vi "Run Framework.vi"(5 "components directory":path, 7 "framework options":T14={"FIFO Options"={"Infinite Timeouts"=FALSE}, "Thread Options"={"Show FP On Call"=TRUE, "Close FP After Call"=TRUE, "Allow Debugging"=TRUE, "Restart On Error"=FALSE}, "Plugin Options"={"Default Components"=TRUE}, "Performance Options"={"Measure Period"=TRUE, "Measure Rx/Tx Duration"=TRUE}}, 8 "error in (no error)":errorcluster, 9 "thread settings":cluster{"Processor":i32, "Priority":i32}={"Processor"=-2, "Priority"=100}, 10 "framework configuration":T2, 11 "user interface pointers (null)":T1) -> (0 "error out":errorcluster)   [LabVIEW 2017]
uses:
  Builds/Data Sharing Framework/Current/Core/DSF Core.lvlibp/Classes/Framework/Framework Options.ctl
  Builds/Data Sharing Framework/Current/Core/DSF Core.lvlibp/Typedefs/DSF FIFO Options.ctl
  Builds/Data Sharing Framework/Current/Core/DSF Core.lvlibp/Classes/Thread/Thread Options.ctl
  Builds/Data Sharing Framework/Current/Core/DSF Core.lvlibp/Typedefs/DSF Plugin Options.ctl
  Builds/Data Sharing Framework/Current/Core/DSF Core.lvlibp/Typedefs/DSF Performance Options.ctl
  Builds/Data Sharing Framework/Current/Core/DSF Core.lvlibp/Typedefs/DSF Engine Framework Configuration.ctl
  Builds/Data Sharing Framework/Current/Core/DSF Core.lvlibp/Typedefs/DSF Engine Plugin Configuration.ctl
  Builds/Data Sharing Framework/Current/Core/DSF Core.lvlibp/Typedefs/DSF Timing Info.ctl
  Builds/Data Sharing Framework/Current/Core/DSF Core.lvlibp/Typedefs/DSF Engine Plugin Thread Configuration.ctl
  Builds/Data Sharing Framework/Current/Core/DSF Core.lvlibp/Typedefs/DSF Settings Info.ctl
  Builds/Data Sharing Framework/Current/Core/DSF Core.lvlibp/Typedefs/DSF Engine Transfer Group Configuration.ctl
  Builds/Data Sharing Framework/Current/Core/DSF Core.lvlibp/Typedefs/DSF Direction.ctl
  Builds/Data Sharing Framework/Current/Core/DSF Core.lvlibp/Typedefs/DSF Engine Transfer Configuration.ctl
  Builds/Data Sharing Framework/Current/Core/DSF Core.lvlibp/Typedefs/DSF Byte Order.ctl
  Builds/Data Sharing Framework/Current/Core/DSF Core.lvlibp/Typedefs/DSF Engine Channel Configuration.ctl
  Builds/Data Sharing Framework/Current/Core/DSF Core.lvlibp/Typedefs/DSF Data Type.ctl
  Builds/Data Sharing Framework/Current/Core/DSF Core.lvlibp/Typedefs/DSF Timeout Behavior.ctl
  SubVIs/UI Pointers.ctl
  <vilib>/NI/Memory Manager/Classes/Pointer/Pointer.lvclass
  <vilib>/NI/Memory Manager/Classes/Pointer/Pointer.lvclass/Pointer.ctl
  <vilib>/Platform/TimedLoop/XDataNode/timing_clust.ctl
  <vilib>/Platform/TimedLoop/XDataNode/nitl_modes.ctl
  <vilib>/Platform/TimedLoop/XDataNode/wakeup.ctl
  <vilib>/NI/Memory Manager/Classes/Pointer/Write U32.vi
  <vilib>/NI/Memory Manager/Classes/Pointer/Read U32.vi
  <vilib>/NI/Memory Manager/Classes/Pointer/Read I32.vi
  <vilib>/NI/Memory Manager/Classes/Pointer/Read Bool.vi
  <vilib>/NI/Memory Manager/Classes/Pointer/Write Bool.vi
  <vilib>/NI/Memory Manager/Classes/Pointer/Write I32.vi
  <vilib>/NI/Memory Manager/Classes/Pointer/Set Address.vi
  <vilib>/NI/Memory Manager/Classes/Pointer/Set Size.vi
  <vilib>/NI/Memory Manager/Classes/Pointer/Set Internal.vi
  <vilib>/NI/Memory Manager/Classes/Pointer/Check Null Pointer.vi
  <vilib>/NI/Memory Manager/Classes/Pointer/Clear (No Check).vi
  <vilib>/NI/Memory Manager/Classes/Pointer/Check Length.vi
  <vilib>/NI/Memory Manager/Classes/Pointer/Write (No Check).vi
  <vilib>/NI/Memory Manager/Classes/Pointer/Write (No Check) U32.vi
  <vilib>/NI/Memory Manager/Classes/Pointer/Check Move.vi
  <vilib>/NI/Memory Manager/Classes/Pointer/Read (No Check).vi
  <vilib>/NI/Memory Manager/Classes/Pointer/Read (No Check) U32.vi
  <vilib>/NI/Memory Manager/Classes/Pointer/Read (No Check) I32.vi
  <vilib>/NI/Memory Manager/Classes/Pointer/Read (No Check) Bool.vi
  <vilib>/NI/Memory Manager/Classes/Pointer/Write (No Check) Bool.vi
  <vilib>/NI/Memory Manager/Classes/Pointer/Write (No Check) I32.vi
  <vilib>/NI/Memory Manager/Classes/Pointer/Get Internal.vi
  <vilib>/NI/Memory Manager/Classes/Pointer/Errors.vi
  <vilib>/NI/Memory Manager/Classes/Pointer/Zone.vi
  <vilib>/NI/Memory Manager/Classes/Pointer/Null Pointer.vi
  <vilib>/NI/Memory Manager/Classes/Pointer/Check Bounds (Pointer).vi
  <vilib>/NI/Memory Manager/Classes/Pointer/Check Count.vi
  <vilib>/NI/Memory Manager/Classes/Pointer/Check Bounds (Power of 2).vi
  <vilib>/NI/Memory Manager/Classes/Pointer/Create Error.vi
  <vilib>/NI/Memory Manager/Classes/Pointer/Out of Bounds.vi
  <vilib>/NI/Memory Manager/Classes/Pointer/Check Bounds.vi
  <vilib>/NI/Memory Manager/Constants/Constants.vi
  <vilib>/NI/Memory Manager/Constants/Library Name.vi
  <vilib>/NI/Memory Manager/Classes/Pointer/Pointer Error Info.vi
  <vilib>/NI/Memory Manager/Constants/Pointer Class Name.vi
  <vilib>/NI/Memory Manager/Classes/Pointer/Write Pointer Size to Error.vi
  <vilib>/NI/Memory Manager/Classes/Pointer/Check Bounds (Buffer).vi
  <vilib>/NI/Memory Manager/Classes/Pointer/Buffer Underflow.vi
  <vilib>/NI/Memory Manager/VIs/New Error Cluster.vi
  <vilib>/NI/Memory Manager/VIs/New Error Cluster (512B).vi
  <vilib>/NI/Memory Manager/VIs/Set Error Status.vi
  <vilib>/NI/Memory Manager/VIs/Set Error Code.vi
  <vilib>/NI/Memory Manager/VIs/Set Error Source.vi
  <vilib>/NI/Memory Manager/VIs/Write String to Source.vi
  <vilib>/NI/Memory Manager/VIs/Write Numeric to Source.vi
  <vilib>/NI/Memory Manager/VIs/Write Numeric Scalar to Source (Base10 U64).vi
  Builds/Data Sharing Framework/Current/Core/DSF Core.lvlibp/Classes/Framework/Framework.lvclass
  <vilib>/platform/TimedLoop/XDataNode/XDataNode.xnode
  <vilib>/Platform/TimedLoop/XDataNode/XDNodeRunTimeDep.lvlib
  Builds/Data Sharing Framework/Current/Core/DSF Core.lvlibp
  Builds/Data Sharing Framework/Current/Core/DSF Core.lvlibp/Classes/Thread/Thread.lvclass
panel:
  out "actual frequency":u32 format="%.0pHz"
  in  "target frequency":u32=100 format="%.0pHz"
  out "iteration":i32
  in  "stop":bool
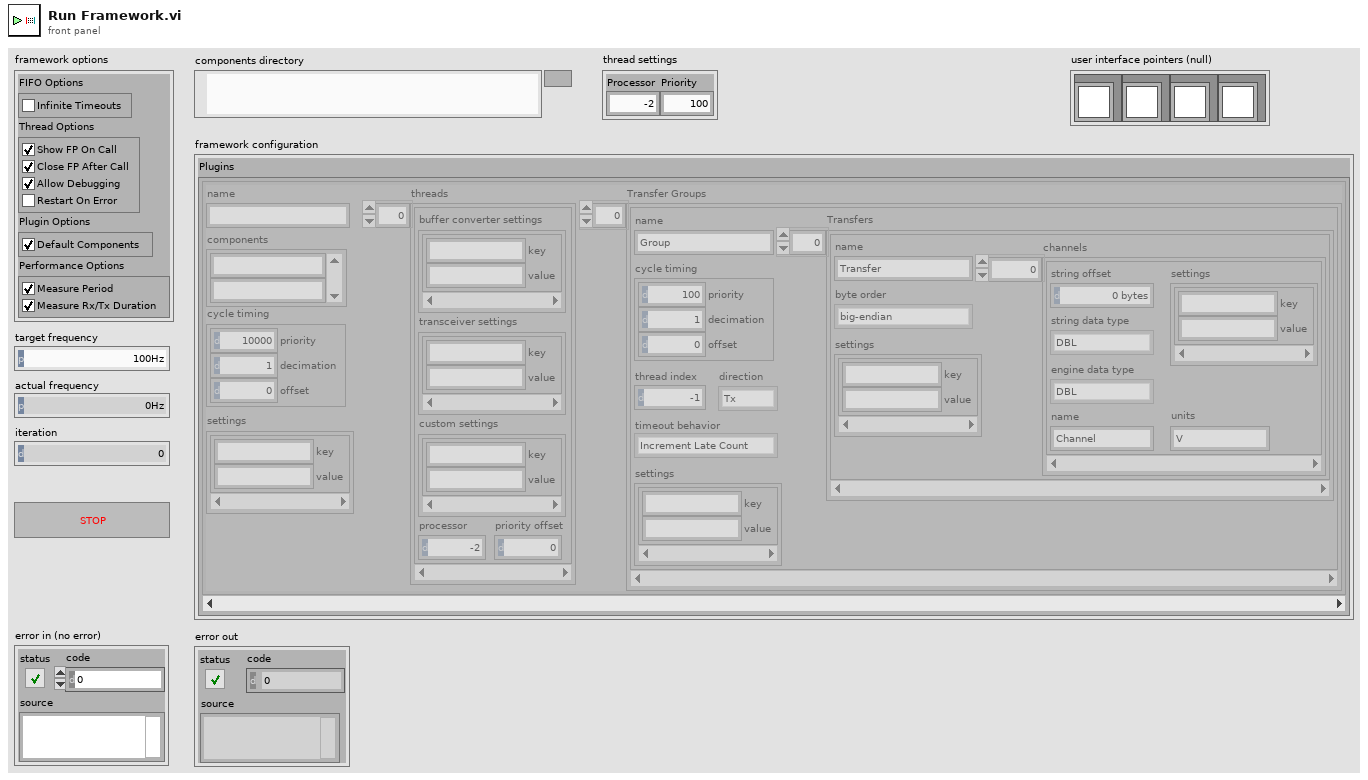
[diagram p1: front panel]
types:
  T1 = typedef "UI Pointers.ctl" = cluster{"Stop":refnum<class "Pointer.lvclass">, "Target Period":refnum<class "Pointer.lvclass">, "Actual Period":refnum<class "Pointer.lvclass">, "Iteration":refnum<class "Pointer.lvclass">}
  T2 = typedef "DSF Core.lvlibp/DSF Engine Framework Configuration.ctl" = cluster{"Plugins":T3[]}
  T3 = typedef "DSF Core.lvlibp/DSF Engine Plugin Configuration.ctl" = cluster{"name":string, "components":string[], "cycle timing":T4, "threads":T5[], "Transfer Groups":T7[], "settings":T6}
  T4 = typedef "DSF Core.lvlibp/DSF Timing Info.ctl" = cluster{"priority":u64, "decimation":u64, "offset":u64}
  T5 = typedef "DSF Core.lvlibp/DSF Engine Plugin Thread Configuration.ctl" = cluster{"buffer converter settings":T6, "transceiver settings":T6, "custom settings":T6, "processor":i32, "priority offset":i16}
  T6 = typedef "DSF Core.lvlibp/DSF Settings Info.ctl" = cluster{"key":string, "value":string}[]
  T7 = typedef "DSF Core.lvlibp/DSF Engine Transfer Group Configuration.ctl" = cluster{"name":string, "direction":T8, "cycle timing":T4, "thread index":i32, "settings":T6, "Transfers":T9[], "timeout behavior":T13}
  T8 = typedef "DSF Core.lvlibp/DSF Direction.ctl" = enum8{"Tx", "Rx"}
  T9 = typedef "DSF Core.lvlibp/DSF Engine Transfer Configuration.ctl" = cluster{"name":string, "byte order":T10, "settings":T6, "channels":T11[]}
  T10 = typedef "DSF Core.lvlibp/DSF Byte Order.ctl" = enum8{"big-endian", "little-endian"}
  T11 = typedef "DSF Core.lvlibp/DSF Engine Channel Configuration.ctl" = cluster{"string offset":u64, "string data type":T12, "engine data type":T12, "name":string, "settings":T6, "units":string}
  T12 = typedef "DSF Core.lvlibp/DSF Data Type.ctl" = enum8{"Bool", "SGL", "DBL", "I8", "I16", "I32", "I64", "U8", "U16", "U32", "U64"}
  T13 = typedef "DSF Core.lvlibp/DSF Timeout Behavior.ctl" = enum8{"Increment Late Count", "Throw Error"}
  T14 = typedef "DSF Core.lvlibp/Framework.lvclass/Framework Options.ctl" = cluster{"FIFO Options":T15, "Thread Options":T16, "Plugin Options":T17, "Performance Options":T18}
  T15 = typedef "DSF Core.lvlibp/Framework.lvclass/DSF FIFO Options.ctl" = cluster{"Infinite Timeouts":bool}
  T16 = typedef "DSF Core.lvlibp/Thread.lvclass/Thread Options.ctl" = cluster{"Show FP On Call":bool, "Close FP After Call":bool, "Allow Debugging":bool, "Restart On Error":bool}
  T17 = typedef "DSF Core.lvlibp/Framework.lvclass/DSF Plugin Options.ctl" = cluster{"Default Components":bool}
  T18 = typedef "DSF Core.lvlibp/DSF Performance Options.ctl" = cluster{"Measure Period":bool, "Measure Rx/Tx Duration":bool}
  T19 = typedef "XDNodeRunTimeDep.lvlib/timing_clust.ctl" = cluster{"Expected End [f-1]":u64, "Actual End [f-1]":u64, "Finished Late? [f-1]":bool, "Expected End [i-1]":u64, "Actual End [i-1]":u64, "Finished Late? [i-1]":bool, "Expected Start [i]":u64, "Actual Start [i]":u64, "Expected Start [f]":u64, "Actual Start [f]":u64, "Source Name":string, "Structure Name":string, "Period":i64, "Deadline":i64, "Offset":i64, "Start":i64, "Priority":i32, "Timeout":i32, "Mode":T20, "Wakeup Reason":T21, "Error":errorcluster, "Source Type":string, "Secondary Source Type":string, "Global End Time":u64, "Global Start Time":u64, "Frame Duration":u64, "Iteration Duration":u64, "Assigned CPU":i32, "I/O Scan Engine Mode":u32}
  T20 = typedef "XDNodeRunTimeDep.lvlib/nitl_modes.ctl" = enum32{"No Change", "Process missed periods, maintain original phase", "Discard missed periods, maintain original phase", "Process missed periods, ignore original phase", "Discard missed periods, ignore original phase"}
  T21 = typedef "XDNodeRunTimeDep.lvlib/wakeup.ctl" = enum32{"Normal", "Aborted", "Asynchronous wakeup", "Timing source error", "Timed loop error", "Timeout"}
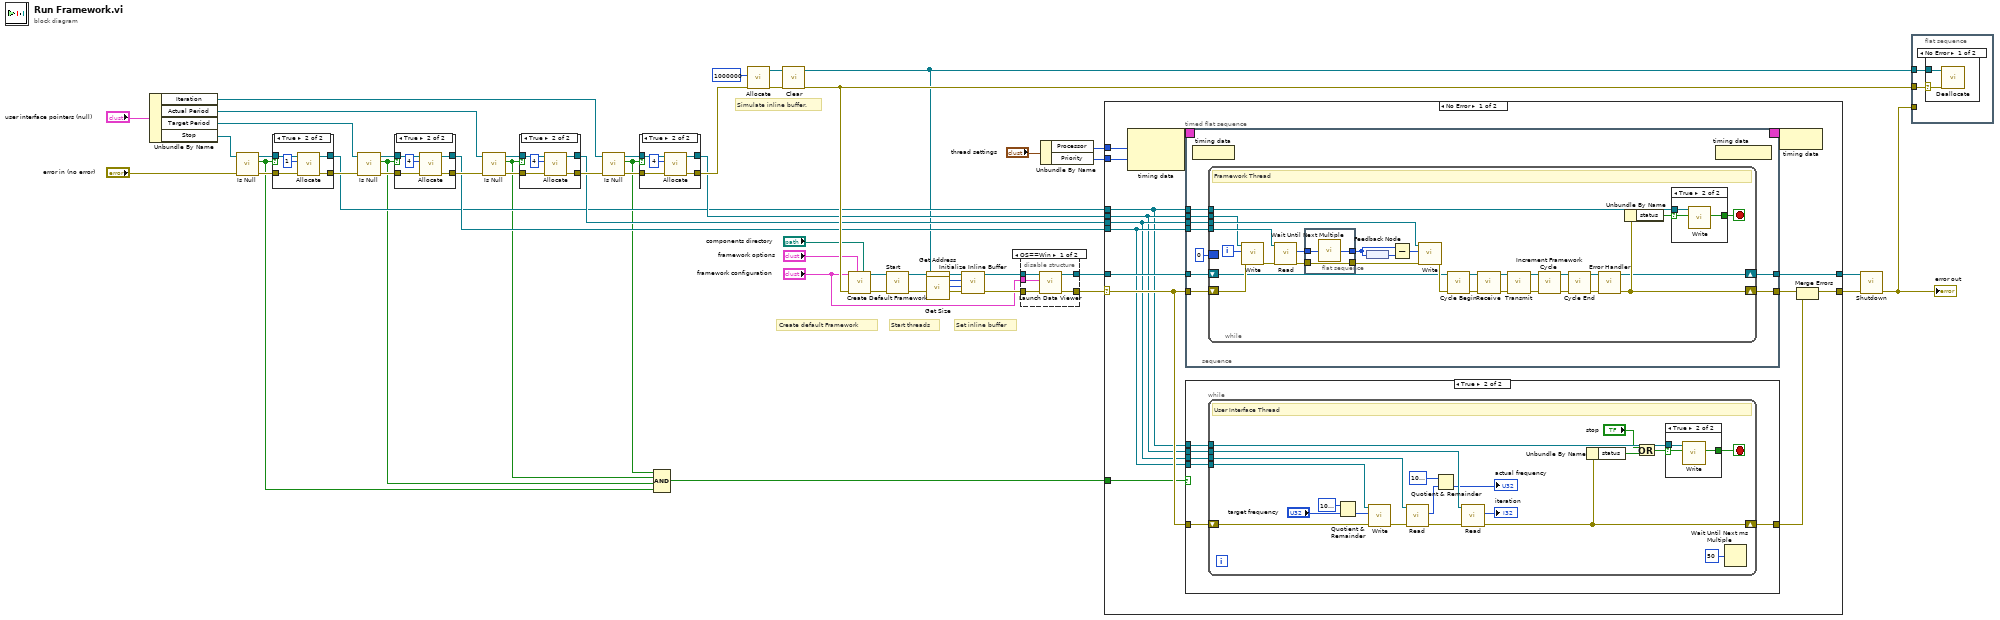
[diagram p0: block diagram]
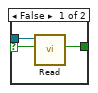
[diagram p5: hidden frame]
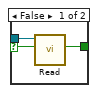
[diagram p6: hidden frame]
diagram:
  # "Set inline buffer"
  # "Start threads"
  # "Create default Framework"
  # "Simulate inline buffer."
  n1 = Unbundle By Name("user interface pointers (null)") -> ("Iteration"=w18:refnum<class "Pointer.lvclass">, "Actual Period"=w22:refnum<class "Pointer.lvclass">, "Target Period"=w26:refnum<class "Pointer.lvclass">, "Stop"=w32:refnum<class "Pointer.lvclass">)
  n2 = call <vilib>:"Is Null.vi"("error in (no error)"="error in (no error)", "Pointer in"=w32) -> ("error out"=w30:errorcluster, "null?"=w5:bool, "Pointer out"=w31:refnum<class "Pointer.lvclass">)  [unwired: 7 in]
  n3 = case shown="True" w5 {
    tunnel: w31 -> [w53 w57]
    tunnel: w30 -> [w52 w56]
    tunnel: [w53 w55] -> w11
    tunnel: [w52 w54] -> w27
    frame False {
    }
    frame True {
      n4 = call <vilib>:"Allocate.vi"("error in (no error)"=w56, "size"=u64 1, "Pointer type"=w57) -> ("error out"=w54:errorcluster, "Pointer out"=w55:refnum<class "Pointer.lvclass">)  [unwired: 7 in]
    }
  }
  n5 = call <vilib>:"Is Null.vi"("error in (no error)"=w27, "Pointer in"=w26) -> ("error out"=w28:errorcluster, "null?"=w4:bool, "Pointer out"=w29:refnum<class "Pointer.lvclass">)  [unwired: 7 in]
  n6 = case shown="True" w4 {
    tunnel: w29 -> [w60 w64]
    tunnel: w28 -> [w59 w63]
    tunnel: [w60 w62] -> w16
    tunnel: [w59 w61] -> w23
    frame False {
    }
    frame True {
      n7 = call <vilib>:"Allocate.vi"("error in (no error)"=w63, "size"=u64 4, "Pointer type"=w64) -> ("error out"=w61:errorcluster, "Pointer out"=w62:refnum<class "Pointer.lvclass">)  [unwired: 7 in]
    }
  }
  n8 = call <vilib>:"Is Null.vi"("error in (no error)"=w23, "Pointer in"=w22) -> ("error out"=w24:errorcluster, "null?"=w3:bool, "Pointer out"=w25:refnum<class "Pointer.lvclass">)  [unwired: 7 in]
  n9 = case shown="True" w3 {
    tunnel: w25 -> [w67 w71]
    tunnel: w24 -> [w66 w70]
    tunnel: [w67 w69] -> w13
    tunnel: [w66 w68] -> w19
    frame False {
    }
    frame True {
      n10 = call <vilib>:"Allocate.vi"("error in (no error)"=w70, "size"=u64 4, "Pointer type"=w71) -> ("error out"=w68:errorcluster, "Pointer out"=w69:refnum<class "Pointer.lvclass">)  [unwired: 7 in]
    }
  }
  n11 = call <vilib>:"Is Null.vi"("error in (no error)"=w19, "Pointer in"=w18) -> ("error out"=w20:errorcluster, "null?"=w2:bool, "Pointer out"=w21:refnum<class "Pointer.lvclass">)  [unwired: 7 in]
  n12 = case shown="True" w2 {
    tunnel: w21 -> [w74 w78]
    tunnel: w20 -> [w73 w77]
    tunnel: [w74 w76] -> w14
    tunnel: [w73 w75] -> w17
    frame False {
    }
    frame True {
      n13 = call <vilib>:"Allocate.vi"("error in (no error)"=w77, "size"=u64 4, "Pointer type"=w78) -> ("error out"=w75:errorcluster, "Pointer out"=w76:refnum<class "Pointer.lvclass">)  [unwired: 7 in]
    }
  }
  n14 = Compound Arithmetic op=AND(w2, w3, w4, w5) -> (w1:bool)
  n15 = call <vilib>:"Allocate.vi"("error in (no error)"=w17, "size"=u64 1000000) -> ("error out"=w46:errorcluster, "Pointer out"=w43:refnum<class "Pointer.lvclass">)  [unwired: 8 in]
  n16 = call <vilib>:"Clear.vi"("error in (no error)"=w46, "Pointer in"=w43) -> ("error out"=w51:errorcluster, "Pointer out"=w10:refnum<class "Pointer.lvclass">)  [unwired: 8 in]
  n17 = call "Create Default Framework.vi"("components directory (default)"="components directory", "framework options"="framework options", "error in (no error)"=w51, "framework configuration"="framework configuration") -> ("error out"=w38:errorcluster, "Framework"=w42:refnum<class "Framework.lvclass">)  [unwired: 6 in]
  n18 = call-dynamic "Start.vi"("error in (no error)"=w38, "Framework in"=w42) -> ("error out"=w41:errorcluster, "Framework out"=w50:refnum<class "Framework.lvclass">)  [unwired: 8 in]
  n19 = call <vilib>:"Get Address.vi"("Pointer in"=w10) -> ("address"=w44:u64)  [unwired: 9 in, 1 out]
  n20 = call <vilib>:"Get Size.vi"("Pointer in"=w10) -> ("size"=w45:u64)  [unwired: 9 in, 1 out]
  n21 = call "Initialize Inline Buffer.vi"("error in (no error)"=w41, "size"=w45, "address"=w44, "Framework in"=w50) -> ("error out"=w39:errorcluster, "Framework out"=w40:refnum<class "Framework.lvclass">)  [unwired: 6 in]
  n22 = disable-structure shown="OS==Win" {
    disable-tunnel: [w84 w86] -> w36
    disable-tunnel: [w83 w85] -> w15
    disable-tunnel: w40 -> [w82 w86]
    disable-tunnel: w39 -> [w81 w85]
    disable-tunnel: "framework configuration" -> [w80 _]
    frame condition #0 (active) {
      n23 = call "Launch Data Viewer.vi"("error in (no error)"=w81, "Framework Configuration"=w80, "Framework in"=w82) -> ("error out"=w83:errorcluster, "Framework out"=w84:refnum<class "Framework.lvclass">)  [unwired: 7 in]
    }
    frame condition #1 {
    }
  }
  n24 = Unbundle By Name("thread settings") -> ("Processor"=w7:i32, "Priority"=w8:i32)
  n25 = case shown="No Error" w15 {
    selector: w15 -> [w101 w197]
    tunnel: [w94 w197] -> w49
    tunnel: w36 -> [w100 w198]
    tunnel: [w98 w198] -> w48
    tunnel: w11 -> [w91 _]
    tunnel: w16 -> [w99 _]
    tunnel: w13 -> [w93 _]
    tunnel: w14 -> [w92 _]
    tunnel: w7 -> [w90 _]
    tunnel: w8 -> [w89 _]
    tunnel: w1 -> [w88 _]
    frame No Error {
      n26 = node-c288(w90, w89) -> (w97:T19)
      n27 = timed-sequence {
        timing: w97 -> [_]
        timing-out: [_] -> w96
        tunnel: w100 -> [w142]
        tunnel: w101 -> [w141]
        tunnel: [w140] -> w98
        tunnel: [w139] -> w95
        tunnel: w91 -> [w138]
        tunnel: w99 -> [w137]
        tunnel: w93 -> [w136]
        tunnel: w92 -> [w135]
        n28 = timed-flat-sequence {
          tunnel: w142 -> [w151]
          tunnel: w141 -> [w150]
          tunnel: [w149] -> w140
          tunnel: [w148] -> w139
          tunnel: w138 -> [w147]
          tunnel: w137 -> [w146]
          tunnel: w136 -> [w145]
          tunnel: w135 -> [w144]
          n29 = node-c288() -> ()  [unwired: 1 in]
          n30 = while {
            shift-right: [w170] -> w149
            shift-left: w151 -> [w155]
            tunnel: w147 -> [w178]
            shift-right: [w173] -> w148
            shift-left: w150 -> [w159]
            tunnel: w146 -> [w171]
            tunnel: w145 -> [w161]
            tunnel: w144 -> [w158]
            border: u32 0 ("Tick Count(uSec)") -> [_]
            i -> [w163]
            stop <- w177 stop-if-true
            # "Framework Thread"
            n31 = call-poly <vilib>:"Write.vi"("error in (no error)"=w159, "value"=w163, "Pointer in"=w158) -> ("error out"=w160:errorcluster)  [unwired: 5 in, 3 out]
            n32 = call-poly <vilib>:"Read.vi"("error in (no error)"=w160, "Pointer in"=w171) -> ("error out"=w157:errorcluster, "value out"=w172:u32)  [unwired: 6 in, 2 out]
            n33 = flat-sequence {
              tunnel: w172 -> [w183]
              tunnel: [w182] -> w154
              tunnel: w157 -> [w181]
              tunnel: [w181] -> w156
              frame #0 {
                n34 = call "Wait Until Next Multiple"("Count(uSec)"=w183) -> ("Tick Count(uSec)"=w182:u32)
              }
            }
            n35 = feedback-in #1(w154) -> ()
            n36 = feedback #1() -> (w152:u32)
            n37 = Subtract(x=w154, y=w152) -> (x-y=w153:u32)
            n38 = call-poly <vilib>:"Write.vi"("error in (no error)"=w156, "value"=w153, "Pointer in"=w161) -> ("error out"=w162:errorcluster)  [unwired: 5 in, 3 out]
            n39 = call "Cycle Begin.vi"("error in (no error)"=w162, "Framework in"=w155) -> ("error out"=w175:errorcluster, "Framework out"=w176:refnum<class "Framework.lvclass">)  [unwired: 8 in]
            n40 = call "Receive.vi"("error in (no error)"=w175, "Framework in"=w176) -> ("error out"=w180:errorcluster, "Framework out"=w179:refnum<class "Framework.lvclass">)  [unwired: 8 in]
            n41 = call "Transmit.vi"("error in (no error)"=w180, "Framework in"=w179) -> ("error out"=w169:errorcluster, "Framework out"=w168:refnum<class "Framework.lvclass">)  [unwired: 8 in]
            n42 = call "Increment Framework Cycle.vi"("error in (no error)"=w169, "Framework in"=w168) -> ("error out"=w166:errorcluster, "Framework out"=w167:refnum<class "Framework.lvclass">)  [unwired: 8 in]
            n43 = call "Cycle End.vi"("error in (no error)"=w166, "Framework in"=w167) -> ("error out"=w165:errorcluster, "Framework out"=w164:refnum<class "Framework.lvclass">)  [unwired: 8 in]
            n44 = call "Error Handler.vi"("error in (no error)"=w165, "Framework in"=w164) -> ("error out"=w173:errorcluster, "Framework out"=w170:refnum<class "Framework.lvclass">)  [unwired: 8 in]
            n45 = Unbundle By Name(w173) -> ("status"=w174:bool)
            n46 = case shown="True" w174 {
              selector: w174 -> [w185 w188]
              tunnel: w178 -> [w186 w189]
              tunnel: [w184 w187] -> w177
              frame False {
                n47 = call-poly <vilib>:"Read.vi"("value in"=w185, "Pointer in"=w186) -> ("value out"=w184:bool)  [unwired: 6 in, 3 out]
              }
              frame True {
                n48 = call-poly <vilib>:"Write.vi"("value"=w188, "Pointer in"=w189) -> ("value"=w187:bool)  [unwired: 6 in, 3 out]
              }
            }
          }
          n49 = node-c288() -> ()  [unwired: 1 out]
        }
      }
      n50 = case shown="True" w88 {
        tunnel: w101 -> [w102 w108]
        tunnel: w99 -> [_ w107]
        tunnel: [w102 w106] -> w87
        tunnel: w93 -> [_ w105]
        tunnel: w92 -> [_ w104]
        tunnel: w91 -> [_ w103]
        frame False {
        }
        frame True {
          n51 = while {
            tunnel: w103 -> [w128]
            shift-right: [w115] -> w106
            shift-left: w108 -> [w123]
            tunnel: w107 -> [w119]
            tunnel: w105 -> [w117]
            tunnel: w104 -> [w113]
            stop <- w127 stop-if-true
            # "User Interface Thread"
            n52 = Quotient & Remainder(x=u32 1000000 ("y"), y="target frequency") -> (floor(x/y)=w118:u32)  [unwired: 1 out]
            n53 = call-poly <vilib>:"Write.vi"("error in (no error)"=w123, "value"=w118, "Pointer in"=w119) -> ("error out"=w120:errorcluster)  [unwired: 5 in, 3 out]
            n54 = call-poly <vilib>:"Read.vi"("error in (no error)"=w120, "Pointer in"=w117) -> ("error out"=w116:errorcluster, "value out"=w109:u32)  [unwired: 6 in, 2 out]
            n55 = Quotient & Remainder(x=u32 1000000 ("y"), y=w109) -> (floor(x/y)=→"actual frequency":u32)  [unwired: 1 out]
            n56 = call-poly <vilib>:"Read.vi"("error in (no error)"=w116, "Pointer in"=w113) -> ("error out"=w115:errorcluster, "value out"=→"iteration":i32)  [unwired: 6 in, 2 out]
            n57 = Unbundle By Name(w115) -> ("status"=w125:bool)
            n58 = Or(x="stop", y=w125) -> (x .or. y?=w126:bool)
            n59 = case shown="True" w126 {
              selector: w126 -> [w130 w133]
              tunnel: w128 -> [w131 w134]
              tunnel: [w129 w132] -> w127
              frame False {
                n60 = call-poly <vilib>:"Read.vi"("value in"=w130, "Pointer in"=w131) -> ("value out"=w129:bool)  [unwired: 6 in, 3 out]
              }
              frame True {
                n61 = call-poly <vilib>:"Write.vi"("value"=w133, "Pointer in"=w134) -> ("value"=w132:bool)  [unwired: 6 in, 3 out]
              }
            }
            n62 = Wait Until Next ms Multiple(millisecond multiple=u32 50) -> ()  [unwired: 1 out]
          }
        }
      }
      n63 = node-c288(w96) -> ()
      n64 = Merge Errors(w95, w87) -> (w94:errorcluster)
    }
    frame Error {
    }
  }
  n65 = call-dynamic "Shutdown.vi"("error in (no error)"=w49, "Framework in"=w48) -> ("error out"=w37:errorcluster)  [unwired: 8 in, 1 out]
  "error out" <- w37
  n66 = flat-sequence {
    tunnel: w10 -> [w200]
    tunnel: w37 -> [_]
    tunnel: w51 -> [w199]
    frame #0 {
      n67 = case shown="No Error" w199 {
        selector: w199 -> [w201 _]
        tunnel: w200 -> [w202 _]
        frame No Error {
          n68 = call <vilib>:"Deallocate.vi"("error in (no error)"=w201, "Pointer"=w202) -> ()  [unwired: 8 in, 2 out]
        }
        frame Error {
        }
      }
    }
  }
